vi "ESA-C Objective Calibration.vi"(2 "Axis":i32=1 min=1 max=3 step=1, 3 "Is Voltage?":bool, 4 "Input Value":dbl) -> (1 "Output Value":dbl)   [LabVIEW 2010]
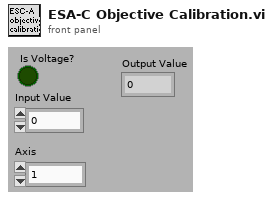
[diagram p1: front panel]
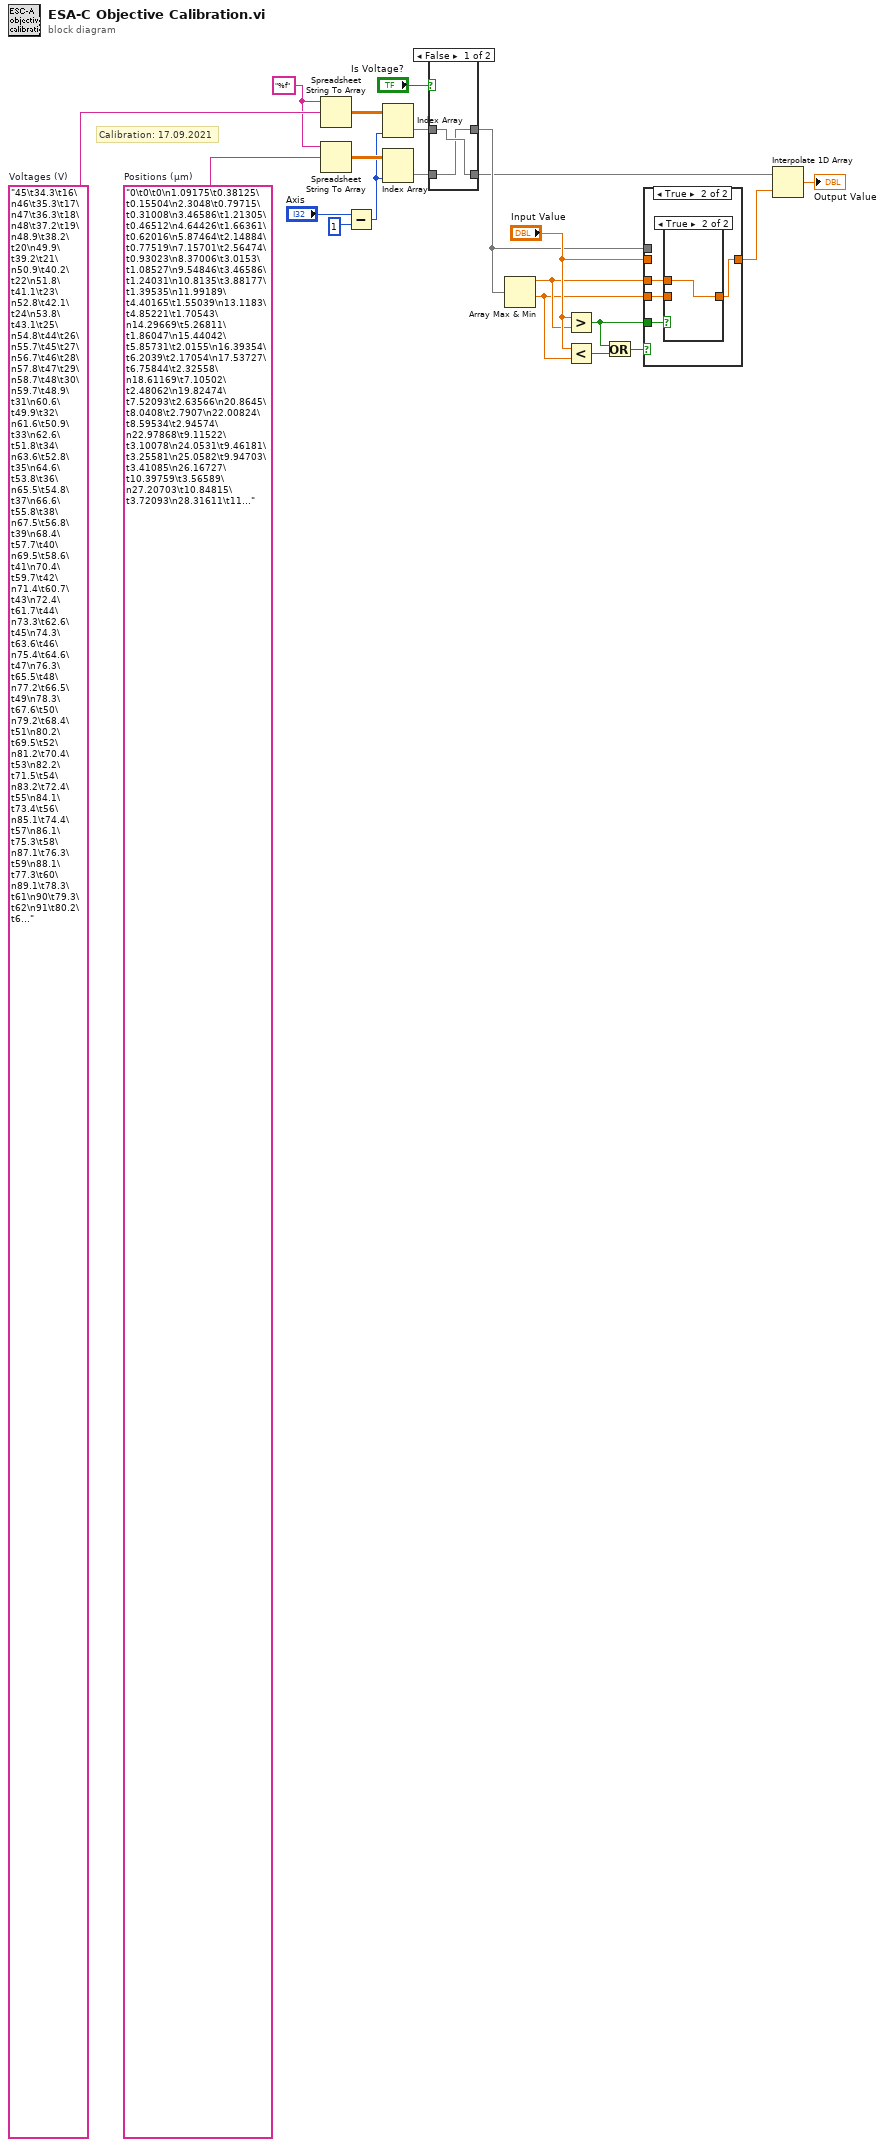
[diagram p0: block diagram]
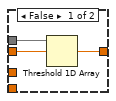
[diagram p2: hidden frame]
diagram:
  w4 = "%f" ("Format-String")
  w6 = "0\t0\t0\n1.09175\t0.38125\t0.15504\n2.3048\t0.79715\t0.31008\n3.46586\t1.21305\t0.46512\n4.64426\t1.66361\t0.62016\n5.87464\t2.14884\t0.77519\n7.15701\t2.56474\t0.93023\n8.37006\t3.0153\t1.08527\n9.54846\t3.46586\t1.24031\n10.8135\t3.88177\t1.39535\n11.99189\t4.40165\t1.55039\n13.1183\t4.85221\t1.70543\n14.29669\t5.26811\t1.86047\n15.44042\t5.85731\t2.0155\n16.39354\t6.2039\t2.17054\n17.53727\t6.75844\t2.32558\n18.61169\t7.10502\t2.48062\n19.82474\t7.52093\t2.63566\n20.8645\t8.0408\t2.7907\n22.00824\t8.59534\t2.94574\n22.97868\t9.11522\t3.10078\n24.0531\t9.46181\t3.25581\n25.0582\t9.94703\t3.41085\n26.16727\t10.39759\t3.56589\n27.20703\t10.84815\t3.72093\n28.31611\t11.33338\t3.87597\n29.32121\t11.78394\t4.03101\n30.32631\t12.30382\t4.18605\n31.40073\t12.6504\t4.34109\n32.37117\t13.13563\t4.49612\n33.48025\t13.55153\t4.65116\n34.48535\t14.00209\t4.8062\n35.55977\t14.45265\t4.96124\n36.42623\t14.8339\t5.11628\n37.46599\t15.2498\t5.27132\n38.36712\t15.75235\t5.42636\n39.40688\t16.16826\t5.5814\n40.308\t16.58416\t5.73643\n41.38242\t16.89609\t5.89147\n42.17957\t17.38131\t6.04651\n43.08069\t17.77988\t6.20155\n44.05113\t18.16113\t6.35659\n44.84828\t18.54237\t6.51163\n45.71475\t18.94095\t6.66667\n46.58121\t19.35685\t6.82171\n47.29172\t19.79008\t6.97674\n48.01955\t20.18866\t7.13178\n48.85135\t20.5699\t7.28682\n49.59652\t20.96848\t7.44186\n50.27236\t21.36705\t7.5969\n51.03485\t21.78296\t7.75194\n51.72802\t22.18153\t7.90698\n52.36921\t22.52812\t8.06202\n53.18369\t22.96135\t8.21705\n53.87686\t23.29061\t8.37209\n54.53537\t23.67185\t8.52713\n55.19389\t23.91446\t8.68217\n55.83507\t24.33037\t8.83721\n56.52824\t24.74627\t8.99225\n56.87483\t25.0582\t9.14729\n57.568\t25.50876\t9.30233\n58.12254\t25.78603\t9.45736\n58.81571\t26.27125\t9.6124\n59.43957\t26.54852\t9.76744\n59.99411\t26.99908\t9.92248\n60.54865\t27.27635\t10.07752\n61.10318\t27.69225\t10.23256\n61.72704\t28.0735\t10.3876\n62.3509\t28.38543\t10.54264\n62.83612\t28.69735\t10.69767\n63.45997\t29.11326\t10.85271\n63.87588\t29.45985\t11.00775\n64.43041\t29.73711\t11.16279\n65.12359\t30.0837\t11.31783\n65.67813\t30.46495\t11.47287\n66.09403\t30.88085\t11.62791\n66.57925\t31.26209\t11.78295\n67.20311\t31.47005\t11.93798\n67.61901\t31.85129\t12.09302\n68.06957\t32.0939\t12.24806\n68.58945\t32.54446\t12.4031\n69.14399\t32.82173\t12.55814\n69.55989\t33.13366\t12.71318\n\t33.41093\t12.86822\n\t33.79218\t13.02326\n\t34.24274\t13.17829\n\t34.45069\t13.33333\n\t34.72796\t13.48837\n\t35.07454\t13.64341\n\t35.42113\t13.79845\n\t35.73306\t13.95349\n\t36.04499\t14.10853\n\t36.42623\t14.26357\n\t36.80748\t14.4186\n\t37.01543\t14.57364\n\t37.39667\t14.72868\n\t37.63928\t14.88372\n\t38.05519\t15.03876\n\t38.22848\t15.1938\n\t38.60973\t15.34884\n\t38.92165\t15.50388\n\t39.23358\t15.65891\n\t39.51085\t15.81395\n\t39.78812\t15.96899\n\t\t16.12403\n\t\t16.27907\n\t\t16.43411\n\t\t16.58915\n\t\t16.74419\n\t\t16.89922\n\t\t17.05426\n\t\t17.2093\n\t\t17.36434\n\t\t17.51938\n\t\t17.67442\n\t\t17.82946\n\t\t17.9845\n\t\t18.13953\n\t\t18.29457\n\t\t18.44961\n\t\t18.60465\n\t\t18.75969\n\t\t18.91473\n\t\t19.06977\n\t\t19.22481\n\t\t19.37984\n\t\t19.53488\n\t\t19.68992\n\t\t19.84496\n\t\t20"  # Positions (µm)
  w5 = "45\t34.3\t16\n46\t35.3\t17\n47\t36.3\t18\n48\t37.2\t19\n48.9\t38.2\t20\n49.9\t39.2\t21\n50.9\t40.2\t22\n51.8\t41.1\t23\n52.8\t42.1\t24\n53.8\t43.1\t25\n54.8\t44\t26\n55.7\t45\t27\n56.7\t46\t28\n57.8\t47\t29\n58.7\t48\t30\n59.7\t48.9\t31\n60.6\t49.9\t32\n61.6\t50.9\t33\n62.6\t51.8\t34\n63.6\t52.8\t35\n64.6\t53.8\t36\n65.5\t54.8\t37\n66.6\t55.8\t38\n67.5\t56.8\t39\n68.4\t57.7\t40\n69.5\t58.6\t41\n70.4\t59.7\t42\n71.4\t60.7\t43\n72.4\t61.7\t44\n73.3\t62.6\t45\n74.3\t63.6\t46\n75.4\t64.6\t47\n76.3\t65.5\t48\n77.2\t66.5\t49\n78.3\t67.6\t50\n79.2\t68.4\t51\n80.2\t69.5\t52\n81.2\t70.4\t53\n82.2\t71.5\t54\n83.2\t72.4\t55\n84.1\t73.4\t56\n85.1\t74.4\t57\n86.1\t75.3\t58\n87.1\t76.3\t59\n88.1\t77.3\t60\n89.1\t78.3\t61\n90\t79.3\t62\n91\t80.2\t63\n92\t81.2\t64\n93\t82.2\t65\n94\t83.2\t66\n95\t84.2\t67\n95.9\t85.1\t68\n96.9\t86.1\t69\n97.9\t87.1\t70\n98.9\t88.1\t71\n99.9\t89.1\t72\n100.8\t90\t73\n101.8\t91\t74\n102.8\t92\t75\n103.8\t93\t76\n104.8\t94\t77\n105.7\t95\t78\n106.7\t96\t79\n107.7\t97\t80\n108.7\t97.9\t81\n109.7\t98.8\t82\n110.7\t99.9\t83\n111.7\t100.8\t84\n112.6\t101.8\t85\n113.6\t102.8\t86\n114.6\t103.8\t87\n115.5\t104.8\t88\n116.6\t105.7\t89\n117.5\t106.7\t90\n118.5\t107.7\t91\n119.5\t108.7\t92\n120.5\t109.7\t93\n121.5\t110.6\t94\n122.5\t111.7\t95\n123.4\t112.6\t96\n124.4\t113.6\t97\n125.4\t114.6\t98\n\t115.6\t99\n\t116.5\t100\n\t117.5\t101\n\t118.6\t102\n\t119.5\t103\n\t120.5\t104\n\t121.4\t105\n\t122.4\t106\n\t123.5\t107\n\t124.4\t108\n\t125.4\t109\n\t126.4\t110\n\t127.4\t111\n\t128.3\t112\n\t129.3\t113\n\t130.3\t114\n\t131.3\t115\n\t132.3\t116\n\t133.2\t117\n\t134.1\t118\n\t135.2\t119\n\t\t120\n\t\t121\n\t\t122\n\t\t123\n\t\t124\n\t\t125\n\t\t126\n\t\t127\n\t\t128\n\t\t129\n\t\t130\n\t\t131\n\t\t132\n\t\t133\n\t\t134\n\t\t135\n\t\t136\n\t\t137\n\t\t138\n\t\t139\n\t\t140\n\t\t141\n\t\t142\n\t\t143\n\t\t144\n\t\t145"  # Voltages (V)
  # "Calibration: 17.09.2021"
  n1 = Spreadsheet String To Array(format string=w4, spreadsheet string=w5) -> (array=w8:dbl[][])  [unwired: 2 in]
  n2 = Spreadsheet String To Array(format string=w4, spreadsheet string=w6) -> (array=w7:dbl[][])  [unwired: 2 in]
  n3 = Subtract(x="Axis", y=1) -> (x-y=w3:i32)
  n4 = Index Array(array=w8, index (col)=w3) -> (element=w12:dbl[])  [unwired: 1 in]
  n5 = Index Array(array=w7, index (col)=w3) -> (element=w13:dbl[])  [unwired: 1 in]
  n6 = case shown="False" "Is Voltage?" {
    tunnel: [w22 w25] -> w20
    tunnel: w12 -> [w23 w25]
    tunnel: [w23 w24] -> w14
    tunnel: w13 -> [w22 w24]
    frame False {
    }
    frame True {
    }
  }
  n7 = Array Max & Min(array=w20) -> (max value=w2:dbl, min value=w1:dbl)  [unwired: 2 out]
  n8 = Greater?(x="Input Value", y=w2) -> (0:w18:bool)
  n9 = Less?(x="Input Value", y=w1) -> (x < y?=w16:bool)
  n10 = Or(x=w18, y=w16) -> (x .or. y?=w17:bool)
  n11 = case shown="True" w17 {
    tunnel: w18 -> [_ w32]
    tunnel: [w26 w31] -> w19
    tunnel: w20 -> [w28 _]
    tunnel: "Input Value" -> [w27 _]
    tunnel: w2 -> [_ w30]
    tunnel: w1 -> [_ w29]
    frame False {
      n12 = Threshold 1D Array(2:w27, 3:w28) -> (0:w26:dbl)  [unwired: 1 in]
    }
    frame True {
      n13 = case shown="True" w32 {
        tunnel: [w33 w34] -> w31
        tunnel: w30 -> [_ w34]
        tunnel: w29 -> [w33 _]
        frame False {
        }
        frame True {
        }
      }
    }
  }
  n14 = Interpolate 1D Array(1:w19, 2:w14) -> (0:→"Output Value":dbl)
